vi "Setup UI.vi"(8 "error in (no error)":errorcluster, 10 "Set UI to input? (F)":bool, 11 "DAQ Digital Code Scan in":refnum<class "DAQ Digital Code Scan.lvclass">) -> (0 "error out":errorcluster, 3 "DAQ Digital Code Scan out":refnum<class "DAQ Digital Code Scan.lvclass">)   [LabVIEW 2012, in "DAQ Digital Code Scan.lvclass"]
doc: "Scanner::Setup is a constructor that has no parameters and faces the user. The Factory calls this VI to let the user configure this Scanner. It is dynamically dispatched in order to let the user choose the type as well as the options of the scanner."
uses:
  DAQ Digital Code Scan.lvclass
  DAQ Digital Code Scan.lvclass/DAQ Digital Code Scan.ctl
panel:
  in  "Send Restart Code":bool
  in  "Next Step Code":i8=2 min=1 step=1
  in  "Reset Code":i8=1 min=1 step=1
  in  "Code On-Time":dbl=0.1
  # "DAQ Digital Scan Setup"
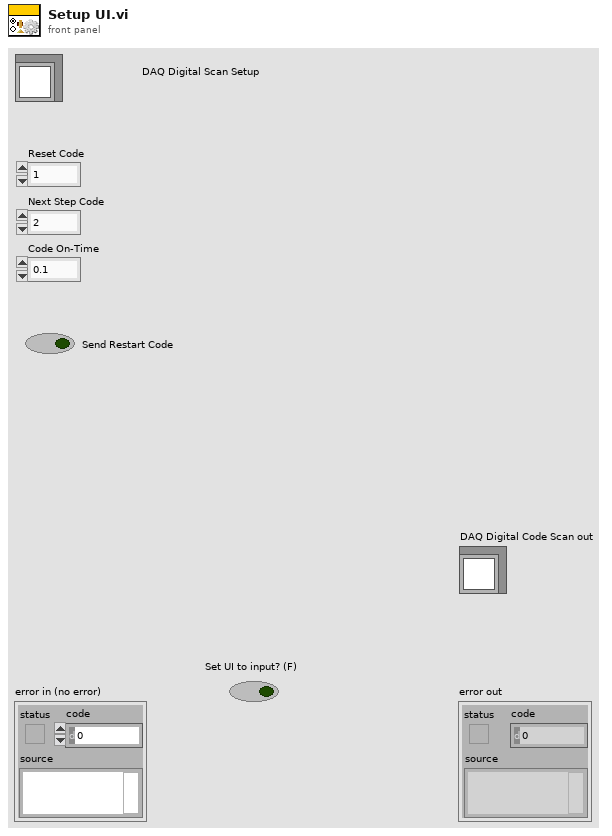
[diagram p1: front panel]
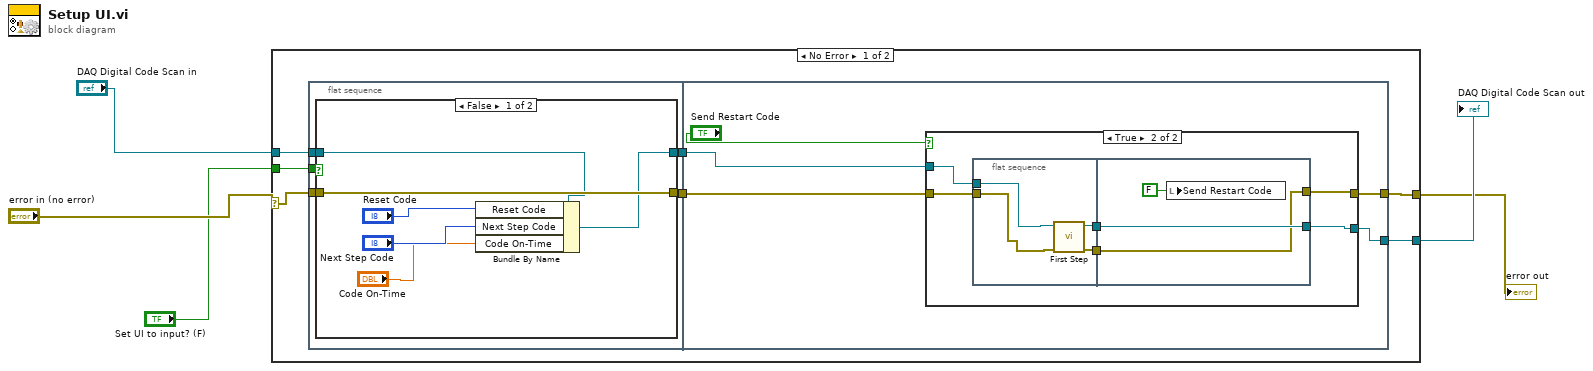
[diagram p0: block diagram]
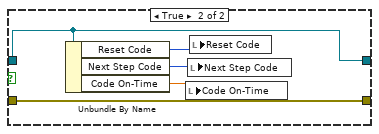
[diagram p2: hidden frame]
diagram:
  n1 = case shown="No Error" "error in (no error)" {
    selector: "error in (no error)" -> [w12 w50]
    tunnel: [w10 w49] -> w4
    tunnel: [w9 w50] -> w2
    tunnel: "DAQ Digital Code Scan in" -> [w8 w49]
    tunnel: "Set UI to input? (F)" -> [w6 _]
    frame No Error {
      n2 = flat-sequence {
        tunnel: w12 -> [w17]
        tunnel: [w16] -> w11
        tunnel: w8 -> [w15]
        tunnel: [w14] -> w7
        tunnel: w6 -> [w13]
        tunnel: w11 -> [w31]
        tunnel: [w33] -> w10
        tunnel: [w32] -> w9
        tunnel: w7 -> [w29]
        frame #0 {
          n3 = case shown="False" w13 {
            tunnel: w17 -> [w23 w28]
            tunnel: [w23 w28] -> w16
            tunnel: w15 -> [w19 w24]
            tunnel: [w18 w24] -> w14
            frame False {
              n4 = Bundle By Name(cluster=w19, "Reset Code"="Reset Code", "Next Step Code"="Next Step Code", "Code On-Time"="Code On-Time") -> (w18:refnum<class "DAQ Digital Code Scan.lvclass">)
            }
            frame True {
              n5 = Unbundle By Name(w24) -> ("Reset Code"=w27:i8, "Next Step Code"=w26:i8, "Code On-Time"=w25:dbl)
              n6 = local write "Code On-Time"(w25) -> ()
              n7 = local write "Next Step Code"(w26) -> ()
              n8 = local write "Reset Code"(w27) -> ()
            }
          }
        }
        frame #1 {
          n9 = case shown="True" "Send Restart Code" {
            tunnel: [w35 w38] -> w32
            tunnel: [w34 w40] -> w33
            tunnel: w31 -> [w35 w37]
            tunnel: w29 -> [w34 w36]
            frame False {
            }
            frame True {
              n10 = flat-sequence {
                tunnel: [w42] -> w41
                tunnel: [w43] -> w39
                tunnel: w37 -> [w44]
                tunnel: w36 -> [w45]
                tunnel: w41 -> [w47]
                tunnel: [w47] -> w40
                tunnel: w39 -> [w46]
                tunnel: [w46] -> w38
                frame #0 {
                  n11 = call-dynamic "First Step.vi"("error in (no error)"=w44, "DAQ Digital Code Scan.lvclass in"=w45) -> ("error out"=w43:errorcluster, "DAQ Digital Code Scan.lvclass out"=w42:refnum<class "DAQ Digital Code Scan.lvclass">)  [unwired: 7 in, 1 out]
                }
                frame #1 {
                  n12 = local write "Send Restart Code"(FALSE ("Send Restart Code")) -> ()
                }
              }
            }
          }
        }
      }
    }
    frame Error {
    }
  }
  "error out" <- w2
  "DAQ Digital Code Scan out" <- w4
